vi "Update Plot Legend and Data Series Names.vi"(8 "error in":errorcluster, 9 "Active Tab":u32, 10 "Page Configurations In":T2(array[cluster]), 11 "XYGraph Ref In":refnum<vi>) -> (0 "error out":errorcluster)   [LabVIEW 2017, in "DTacq Plot Display Library.lvlib"]
doc: "Updates the plot area, to match the settings for the currently selected tab.\n\nUpdates the plot area to;\n-Have the correct number of data series for this tab\n -Set the data series names and colours\n-Have a plot legend of appropriate size"
uses:
  DTacq Plot Display Library.lvlib
  Typedefs/Plot Channel Configruation--Cluster.ctl
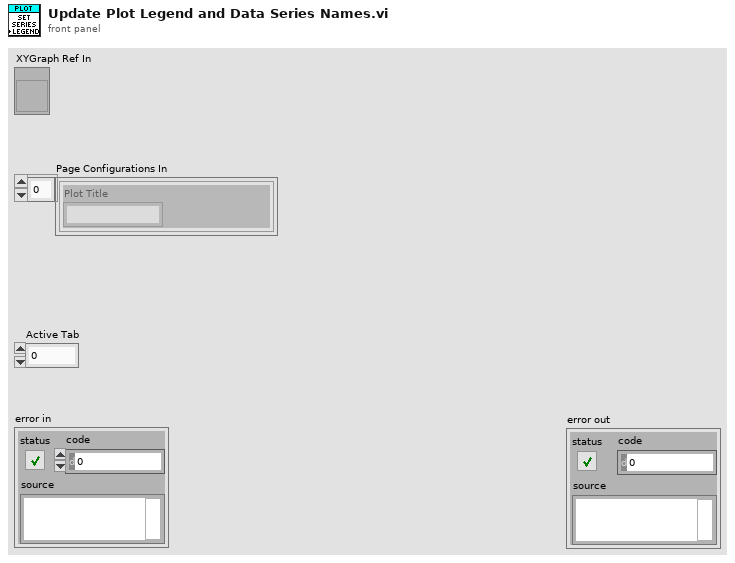
[diagram p1: front panel]
types:
  T1 = typedef "DTacq Plot Display Library.lvlib/Plot Channel Configruation--Cluster.ctl" = cluster{"Shared Variable Reference":refnum<k21>, "Full Variable Name":string, "URL":string, "Descriptive Name":string, "Data Type":variant, "Colour":u32}
  T2 = cluster{"Plot Title":string, "Y-Axis Label":string, "X-Axis Label":string, "Plot Channel Configurations":T1[]}[]
  T3 = cluster{"Plot Title":string, "Y-Axis Label":string, "X-Axis Label":string, "Plot Channel Configurations":T1[]}
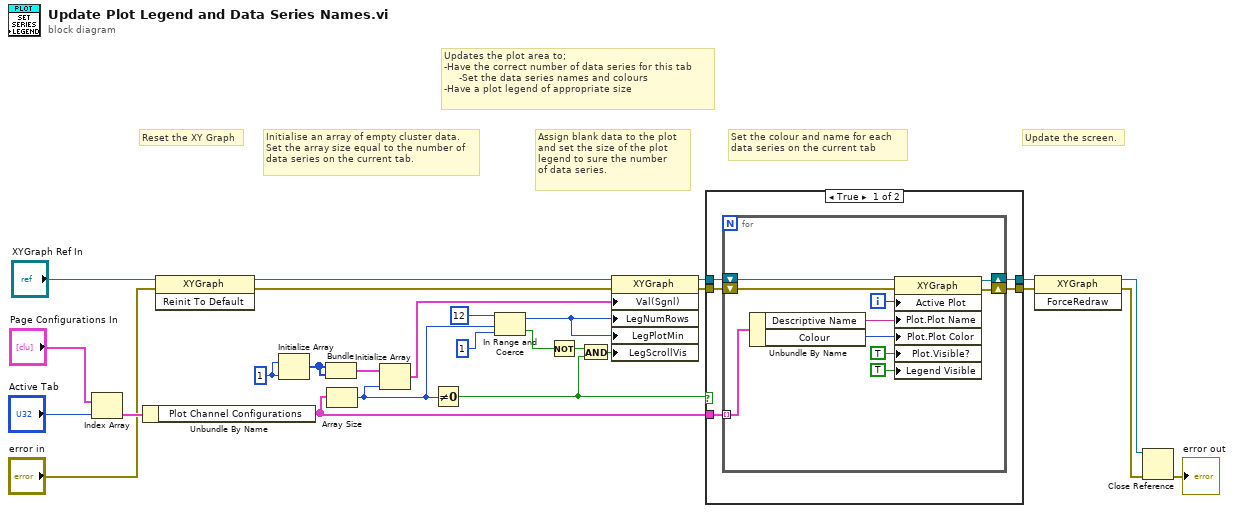
[diagram p0: block diagram]
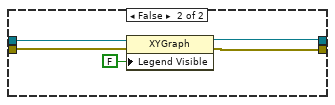
[diagram p2: hidden frame]
diagram:
  w24 = 1 ("dimension size")
  # "Updates the plot area to;\n-Have the correct number of data series for this tab\n     -Set the data series names and colours\n-Have a plot legend of appropriate size"
  # "Update the screen."
  # "Set the colour and name for each\ndata series on the current tab"
  # "Assign blank data to the plot\nand set the size of the plot\nlegend to sure the number\nof data series."
  # "Initialise an array of empty cluster data.\nSet the array size equal to the number of\ndata series on the current tab."
  # "Reset the XY Graph"
  n1 = Index Array(array="Page Configurations In", index="Active Tab") -> (element=w26:T3)
  n2 = Unbundle By Name(w26) -> ("Plot Channel Configurations"=w20:T1[])
  n3 = invoke class="XYGraph" method="Reinit To Default"(reference="XYGraph Ref In", error in="error in") -> (reference out=w13:refnum<vi>, error out=w12:errorcluster)  [unwired: 1 in, 1 out]
  n4 = Initialize Array(w24, w24) -> (w21:i32[])
  n5 = Bundle(w21, w21) -> (w23:cluster{i32[], i32[]})  [unwired: 1 in]
  n6 = Array Size(array=w20) -> (size(s)=w8:i32)
  n7 = Initialize Array(w23, w8) -> (w22:cluster{i32[], i32[]}[])
  n8 = Not Equal To 0?(x=w8) -> (x != 0?=w4:bool)
  n9 = In Range and Coerce(upper limit=i16 12, x=w8, lower limit=i16 1) -> (coerced(x)=w1:i32, In Range?=w3:bool)
  n10 = Not(x=w3) -> (.not. x?=w2:bool)
  n11 = And(x=w2, y=w4) -> (x .and. y?=w5:bool)
  n12 = property class="XYGraph"(reference=w13, error in=w12, "Val(Sgnl)"=w22, "LegNumRows"=w1, "LegPlotMin"=w1, "LegScrollVis"=w5) -> (reference out=w15:refnum<vi>, error out=w11:errorcluster)
  n13 = case shown="True" w4 {
    tunnel: w20 -> [w32 _]
    tunnel: [w31 w45] -> w19
    tunnel: [w30 w44] -> w17
    tunnel: w15 -> [w29 w47]
    tunnel: w11 -> [w28 w46]
    frame True {
      n14 = for {
        tunnel: w32 -> [w40] mode=indexing
        shift-right: [w37] -> w31
        shift-left: w29 -> [w42]
        shift-right: [w36] -> w30
        shift-left: w28 -> [w35]
        i -> [w41]
        n15 = Unbundle By Name(w40) -> ("Descriptive Name"=w39:string, "Colour"=w38:u32)
        n16 = property class="XYGraph"(reference=w42, error in=w35, "Active Plot"=w41, "Plot.Plot Name"=w39, "Plot.Plot Color"=w38, "Plot.Visible?"=TRUE ("Plot.Visible"), "Legend Visible"=TRUE ("Legend:Disable")) -> (reference out=w37:refnum<vi>, error out=w36:errorcluster)
      }
    }
    frame False {
      n17 = property class="XYGraph"(reference=w47, error in=w46, "Legend Visible"=FALSE ("Legend:Disable")) -> (reference out=w45:refnum<vi>, error out=w44:errorcluster)
    }
  }
  n18 = invoke class="XYGraph" method="ForceRedraw"(reference=w19, error in=w17) -> (reference out=w18:refnum<vi>, error out=w16:errorcluster)  [unwired: 1 in, 1 out]
  n19 = Close Reference(reference=w18, error in (no error)=w16) -> (error out=→"error out":errorcluster)
